vi "TEST_Write Query and Results TDM.vi"() -> ()   [LabVIEW 2011]
uses:
  Datafinder Query.ctl
  eSearch Types.ctl
  DataFinder Comparisons.ctl
  <vilib>/Platform/storage/Storage.llb/usiSequenceRepresentation.ctl
  <vilib>/Platform/storage/lvStorage.llb/_openStorageWithRootAutoDetect.vi
  <vilib>/Platform/storage/lvStorage.llb/xStorage/xStorageSupp/ErrorOut.vi
  <vilib>/Platform/storage/lvStorage.llb/_createOrGetByNameExplicitChildObject.vi
  <vilib>/Platform/storage/Storage.llb/__savePropString.vi
  <vilib>/Platform/storage/lvStorage.llb/_saveStringChannel.vi
  <vilib>/Platform/storage/Storage.llb/Get Object Info.vi
  <vilib>/Platform/storage/Storage.llb/__closeStorageFromObject.vi
  <vilib>/Platform/storage/lvStorage.llb/xStorage/Open Data Storage/Open Data Storage.xnode
  <vilib>/Platform/storage/lvStorage.llb/xStorage/Write Data/Write Data.xnode
  <vilib>/Platform/storage/lvStorage.llb/xStorage/Close Data Storage/Close Data Storage.xnode
panel:
  out "Results Array":string[][](array[string])
  out "Condition Array":string[][](array[string])
  in  "Return Type (ChannelGroup)":T1=enum."eSearchChannelGroup"
  in  "DataFinder parameters":T2[](array[typedef])
  out "error out":errorcluster
  in  "error in (no error)":errorcluster
  in  "Query Path":path=path "I:/Engineering/Development/SPARTAN/www/cgi-bin/cgi-lib/Database/Datafinder/test2.tdm"
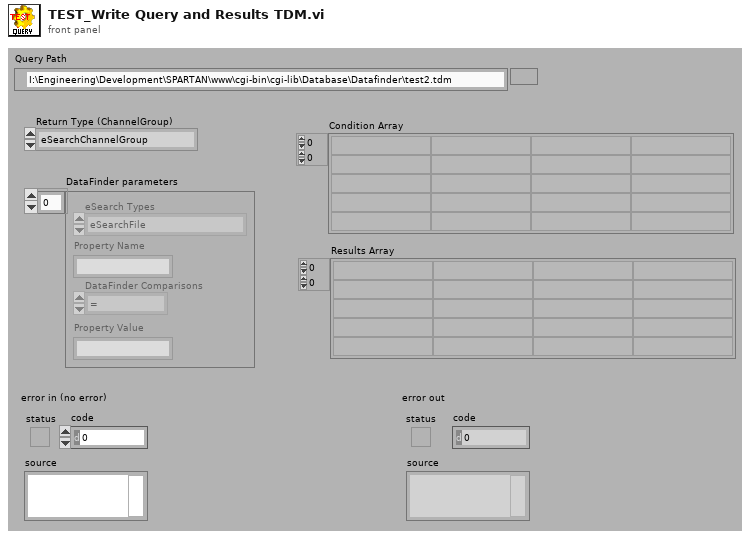
[diagram p1: front panel]
types:
  T1 = typedef "eSearch Types.ctl" = enum16{"eSearchFile", "eSearchChannelGroup", "eSearchChannel"}
  T2 = typedef "Datafinder Query.ctl" = cluster{"eSearch Types":T1, "Property Name":string, "DataFinder Comparisons":T3, "Property Value":string}
  T3 = typedef "DataFinder Comparisons.ctl" = enum16{"=", "<>", "<", "<=", ">", ">="}
  T4 = enum16{"open", "open or create", "create or replace", "create", "open (read only)"}
  T5 = enum16{"UPDATE", "READ", "QUERY", "CREATE CHILD", "CREATE", "CONNECT", "DISCONNECT"}
  T6 = enum16{"Append values", "Replace values at index", "Replace all values"}
  T7 = typedef "usiSequenceRepresentation.ctl" = enum16{"explicit", "implicit"}
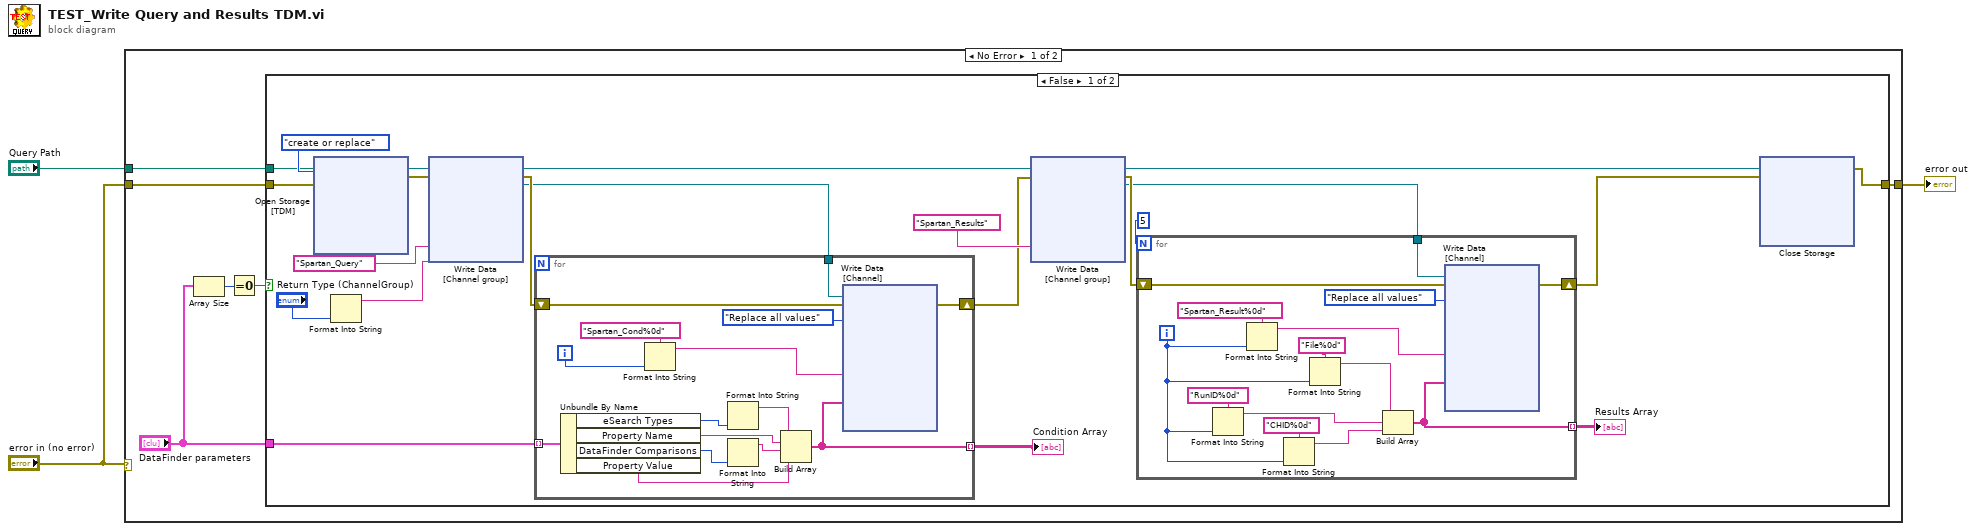
[diagram p0: block diagram]
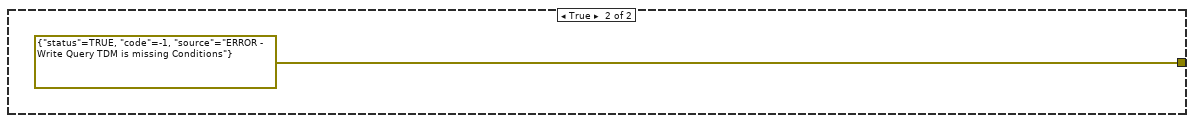
[diagram p2: hidden frame]
diagram:
  n1 = case shown="No Error" "error in (no error)" {
    tunnel: "Query Path" -> [w9 _]
    tunnel: "error in (no error)" -> [w8 w162]
    tunnel: [w7 w162] -> w1
    frame No Error {
      n2 = Array Size(array="DataFinder parameters") -> (size(s)=w5:i32)
      n3 = Equal To 0?(x=w5) -> (x = 0?=w4:bool)
      n4 = case shown="False" w4 {
        tunnel: w9 -> [w25 _]
        tunnel: w8 -> [w24 _]
        tunnel: "DataFinder parameters" -> [w23 _]
        tunnel: [w21 errorcluster {"status"=TRUE, "code"=-1, "source"="ERROR - Write Query TDM is missing Conditions"} ("error out")] -> w7
        frame False {
          n5 = xnode "Open Storage\n[TDM]"("file path"=w25, "function (open:0)"=T4."create or replace", "error in (no error)"=w24) -> ("storage refnum (file)"=w31:refnum<k20>, "error out"=w29:errorcluster)  [unwired: 2 in, 1 out]
          n6 = Format Into String("Return Type (ChannelGroup)") -> (resulting string=w22:string)  [unwired: 3 in, 1 out]
          n7 = xnode "Write Data\n[Channel group]"("Name"="Spartan_Query", "Description"=w22, "storage refnum (file)"=w31, "error in"=w29) -> ("storage refnum (file) out"=w18:refnum<k20>, "error out"=w28:errorcluster, "storage refnum (channel group)"=w27:refnum<k20>)
          n8 = for {
            tunnel: w27 -> [w134]
            shift-right: [w133] -> w15
            shift-left: w28 -> [w136]
            tunnel: w23 -> [w132] mode=indexing
            tunnel: [w122] -> w19 mode=indexing
            i -> [w124]
            n9 = Unbundle By Name(w132) -> ("eSearch Types"=w131:T1, "Property Name"=w129:string, "DataFinder Comparisons"=w128:T3, "Property Value"=w126:string)
            n10 = Format Into String(format string="Spartan_Cond%0d", w124) -> (resulting string=w123:string)  [unwired: 2 in, 1 out]
            n11 = Format Into String(w131) -> (resulting string=w130:string)  [unwired: 3 in, 1 out]
            n12 = Format Into String(w128) -> (resulting string=w127:string)  [unwired: 3 in, 1 out]
            n13 = Build Array(w130, w129, w127, w126) -> (w122:string[])
            n14 = xnode "Write Data\n[Channel]"("Name"=w123, "Signal"=w122, "storage refnum (channel group)"=w134, "error in"=w136, "append / replace (append data values)"=T6."Replace all values") -> ("error out"=w133:errorcluster)  [unwired: 4 out]
          }
          "Condition Array" <- w19
          n15 = xnode "Write Data\n[Channel group]"("Name"="Spartan_Results", "storage refnum (file)"=w18, "error in"=w15) -> ("storage refnum (file) out"=w12:refnum<k20>, "error out"=w14:errorcluster, "storage refnum (channel group)"=w11:refnum<k20>)  [unwired: 1 out]
          n16 = for {
            N: 5 -> [_]
            shift-right: [w95] -> w13
            shift-left: w14 -> [w97]
            tunnel: [w92] -> w16 mode=indexing
            tunnel: w11 -> [w84]
            i -> [w86]
            n17 = Format Into String(format string="RunID%0d", w86) -> (resulting string=w89:string)  [unwired: 2 in, 1 out]
            n18 = Format Into String(format string="Spartan_Result%0d", w86) -> (resulting string=w93:string)  [unwired: 2 in, 1 out]
            n19 = Format Into String(format string="CHID%0d", w86) -> (resulting string=w85:string)  [unwired: 2 in, 1 out]
            n20 = Format Into String(format string="File%0d", w86) -> (resulting string=w90:string)  [unwired: 2 in, 1 out]
            n21 = Build Array(w90, w89, w85) -> (w92:string[])
            n22 = xnode "Write Data\n[Channel]"("Name"=w93, "Signal"=w92, "storage refnum (channel group)"=w84, "error in"=w97, "append / replace (append data values)"=T6."Replace all values") -> ("error out"=w95:errorcluster)  [unwired: 4 out]
          }
          "Results Array" <- w16
          n23 = xnode "Close Storage\n"("storage refnum (file)"=w12, "error in (no error)"=w13) -> ("error out"=w21:errorcluster)  [unwired: 1 out]
        }
        frame True {
        }
      }
    }
    frame Error {
    }
  }
  "error out" <- w1
